vi "GetAttributes__slk_msxml.vi"(0 "document in":refnum<class "msxml document.lvclass">, 5 "node in":refnum<class "msxml node.lvclass">, 11 "error in (no error)":errorcluster) -> (4 "document out":refnum<class "msxml document.lvclass">, 6 "node out":refnum<class "msxml node.lvclass">, 14 "attributes":T1, 15 "error out":errorcluster)   [LabVIEW 2020, in "MSXML.lvlib" / "msxml node.lvclass"]
doc: "Returns the attributes value of MSXML Node."
uses:
  msxml node.lvclass
  MSXML Document/msxml document.lvclass
  Type Definition/Attributes__slk_msxml.ctl
  Type Definition/Attribute__slk_msxml.ctl
  msxml node.lvclass/msxml node.ctl
  MSXML.lvlib
panel:
  # "GetAttributes__slk_msxml.vi\n\nReturns the attributes value of MSXML Node.\n\nNOTICE -- YOU MUST LEAVE THIS NOTICE IN PLACE.\n\nCopyright (c) 2004-2010 Shawn Liu <shawn.liu.cn@gmail.com>\n\nAll rights reserved."
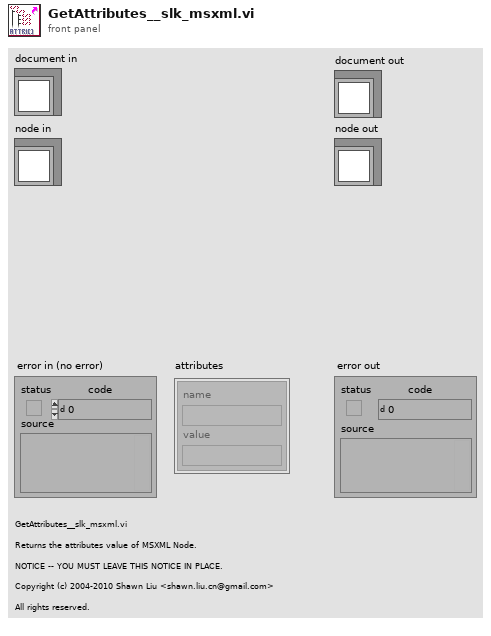
[diagram p1: front panel]
types:
  T1 = typedef "MSXML.lvlib/Attributes__slk_msxml.ctl" = T2[]
  T2 = typedef "MSXML.lvlib/Attribute__slk_msxml.ctl" = cluster{"name":string, "value":string}
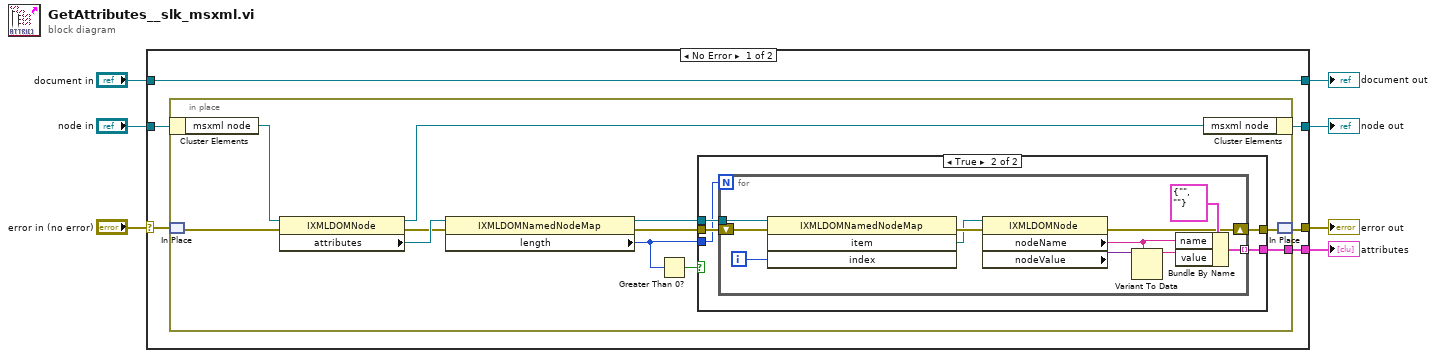
[diagram p0: block diagram]
diagram:
  n1 = case shown="No Error" "error in (no error)" {
    selector: "error in (no error)" -> [w13 w44]
    tunnel: [w12 w44] -> w4
    tunnel: [w10 w43] -> w6
    tunnel: "node in" -> [w11 w43]
    tunnel: [w9 _] -> w3
    tunnel: "document in" -> [w8 w42]
    tunnel: [w8 w42] -> w1
    frame No Error {
      n2 = in-place {
        in-place-border: [w15] -> w9
        n3 = in-place-cluster #1(w11) -> ("msxml node"=w24:refnum<k7>)
        n4 = in-place-match #2(w13) -> (w22:errorcluster)
        n5 = property class="IXMLDOMNode"(reference=w24, error in=w22) -> (reference out=w20:refnum<k7>, error out=w21:errorcluster, "attributes"=w23:refnum<k7>)
        n6 = property class="IXMLDOMNamedNodeMap"(reference=w23, error in=w21) -> (reference out=w16:refnum<k7>, error out=w19:errorcluster, "length"=w17:i32)
        n7 = Greater Than 0?(x=w17) -> (x > 0?=w18:bool)
        n8 = case shown="True" w18 {
          tunnel: w19 -> [w25 w29]
          tunnel: w17 -> [_ w28]
          tunnel: w16 -> [_ w30]
          tunnel: [_ w27] -> w15
          tunnel: [w25 w26] -> w14
          frame False {
          }
          frame True {
            n9 = for {
              N: w28 -> [_]
              tunnel: w30 -> [w39]
              shift-right: [w33] -> w26
              shift-left: w29 -> [w32]
              tunnel: [w31] -> w27 mode=indexing
              i -> [w38]
              n10 = invoke class="IXMLDOMNamedNodeMap" method="item"(reference=w39, error in=w32, "index"=w38) -> (error out=w41:errorcluster, "item"=w40:refnum<k7>)  [unwired: 1 in, 2 out]
              n11 = property class="IXMLDOMNode"(reference=w40, error in=w41) -> (error out=w33:errorcluster, "nodeName"=w34:string, "nodeValue"=w36:variant)  [unwired: 1 out]
              n12 = Variant To Data(type=w34, Variant=w36) -> (data=w35:string)  [unwired: 1 in, 1 out]
              n13 = Bundle By Name(cluster=T2 {"name"="", "value"=""} ("attribute"), "name"=w34, "value"=w35) -> (w31:T2)
            }
          }
        }
        n14 = in-place-cluster #1("msxml node"=w20) -> (w10:refnum<class "msxml node.lvclass">)
        n15 = in-place-match #2(w14) -> (w12:errorcluster)
      }
    }
    frame Error {
    }
  }
  "node out" <- w6
  "error out" <- w4
  "attributes" <- w3
  "document out" <- w1
